vi "SpeedTest.vi"() -> ()   [LabVIEW 2010]
panel:
  out "Numeric":i32
  out "x/y":dbl
  in  "Vi to open":enum16{"JILTest", "JILTest2", "JILTestR"}(ring)
  in  "stringin":string
  in  "booleanin":bool=TRUE
  in  "doublein":dbl
  in  "intin":i32
  in  "Mensajes":T1(ring)
  in  "stop":bool
  in  "Send":bool=TRUE
  out "error out":errorcluster
  out "Respuesta":string
  out "Mensaje":string
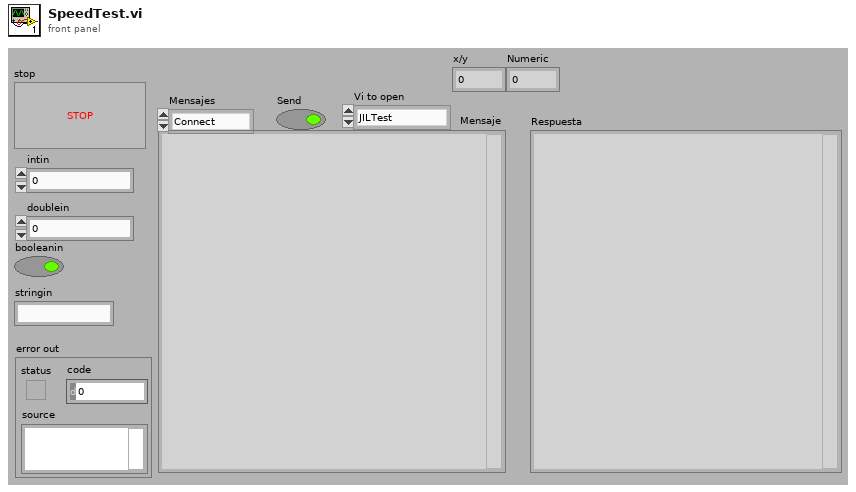
[diagram p1: front panel]
types:
  T1 = enum16{"Connect", "OpenVi", "SyncVi", "RunVi", "StopVi", "CloseVi", "Disconnect"}
  T2 = enum16{"Standard", "Buffered", "CRLF", "Immediate"}
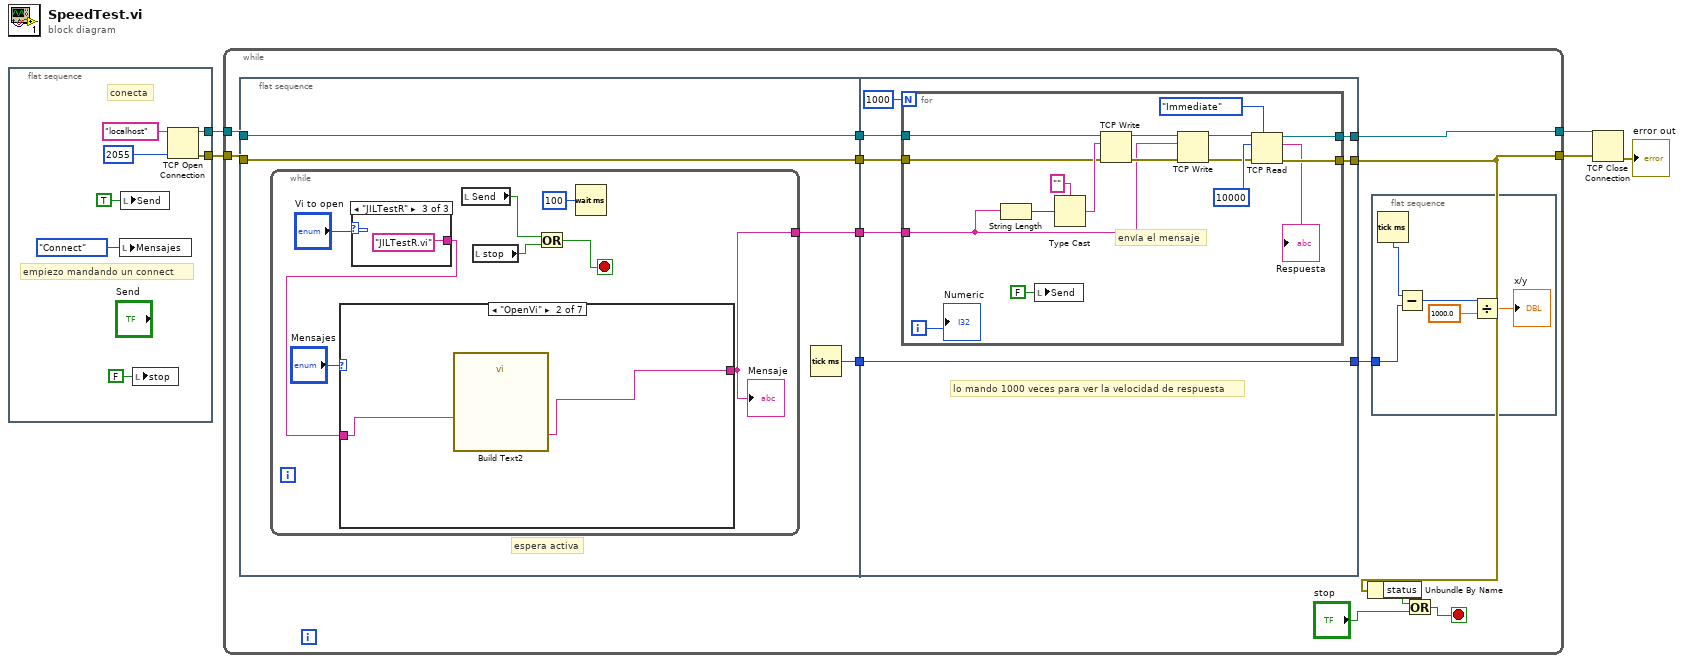
[diagram p0: block diagram]
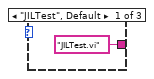
[diagram p2: hidden frame]
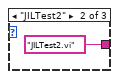
[diagram p3: hidden frame]
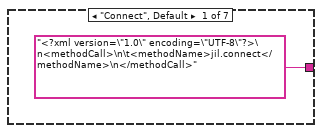
[diagram p4: hidden frame]
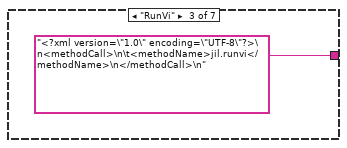
[diagram p5: hidden frame]
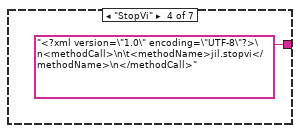
[diagram p6: hidden frame]
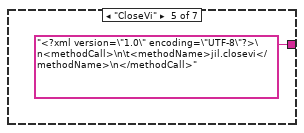
[diagram p7: hidden frame]
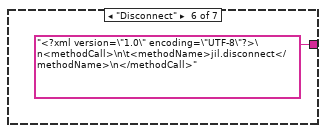
[diagram p8: hidden frame]
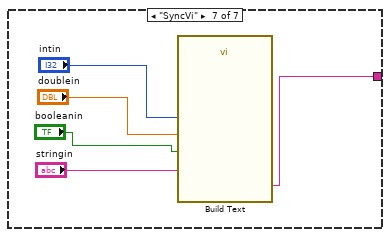
[diagram p9: hidden frame]
diagram:
  n1 = flat-sequence {
    tunnel: [w10] -> w5
    tunnel: [w9] -> w4
    frame #0 {
      # "empiezo mandando un connect"
      # "conecta"
      n2 = local write "Mensajes"(T1."Connect" ("Mensajes")) -> ()
      n3 = local write "Send"(TRUE ("Send")) -> ()
      n4 = local write "stop"(FALSE ("stop")) -> ()
      n5 = TCP Open Connection(address="localhost", remote port or service name=u16 2055) -> (connection ID=w10:refnum<k5>, error out=w9:errorcluster)  [unwired: 3 in]
    }
  }
  n6 = while {
    tunnel: w5 -> [w22]
    tunnel: w4 -> [w21]
    tunnel: [w20] -> w2
    tunnel: [w17] -> w1
    stop <- w18 stop-if-true
    n7 = flat-sequence {
      tunnel: [w33] -> w24
      tunnel: [w32] -> w23
      tunnel: [w31] -> w15
      tunnel: w21 -> [w33]
      tunnel: w22 -> [w32]
      tunnel: [w30] -> w14
      tunnel: [w63] -> w20
      tunnel: [w62] -> w17
      tunnel: w24 -> [w61]
      tunnel: w23 -> [w60]
      tunnel: w15 -> [w59]
      tunnel: [w58] -> w13
      tunnel: w14 -> [w58]
      frame #0 {
        # "espera activa"
        n8 = while {
          tunnel: [w36] -> w31
          stop <- w40 stop-if-true
          n9 = case shown="\"JILTestR\"" "Vi to open" {
            tunnel: ["JILTest.vi" "JILTest2.vi" "JILTestR.vi"] -> w34
            frame "JILTest", Default {
            }
            frame "JILTest2" {
            }
            frame "JILTestR" {
            }
          }
          n10 = case shown="\"OpenVi\"" "Mensajes" {
            tunnel: ["<?xml version=\"1.0\" encoding=\"UTF-8\"?>\n<methodCall>\n\t<methodName>jil.connect</methodName>\n</methodCall>" w46 "<?xml version=\"1.0\" encoding=\"UTF-8\"?>\n<methodCall>\n\t<methodName>jil.runvi</methodName>\n</methodCall>\n" "<?xml version=\"1.0\" encoding=\"UTF-8\"?>\n<methodCall>\n\t<methodName>jil.stopvi</methodName>\n</methodCall>" "<?xml version=\"1.0\" encoding=\"UTF-8\"?>\n<methodCall>\n\t<methodName>jil.closevi</methodName>\n</methodCall>" "<?xml version=\"1.0\" encoding=\"UTF-8\"?>\n<methodCall>\n\t<methodName>jil.disconnect</methodName>\n</methodCall>" w56] -> w36
            tunnel: w34 -> [_ w47 _ _ _ _ _]
            frame "Connect", Default {
            }
            frame "OpenVi" {
              n11 = call "Build Text2"("name"=w47) -> ("Result"=w46:string)  [unwired: 13 in, 1 out]
            }
            frame "RunVi" {
            }
            frame "StopVi" {
            }
            frame "CloseVi" {
            }
            frame "Disconnect" {
            }
            frame "SyncVi" {
              n12 = call "Build Text"("string"="stringin", "int"="intin", "double"="doublein", "bolean"="booleanin") -> ("Result"=w56:string)  [unwired: 10 in, 1 out]
            }
          }
          "Mensaje" <- w36
          n13 = local read "Send"() -> (w38:bool)
          n14 = local read "stop"() -> (w39:bool)
          n15 = Or(x=w38, y=w39) -> (x .or. y?=w40:bool)
          n16 = Wait (ms)(milliseconds to wait=u32 100) -> ()  [unwired: 1 out]
        }
        n17 = Tick Count (ms)() -> (millisecond timer value=w30:u32)
      }
      frame #1 {
        # "lo mando 1000 veces para ver la velocidad de respuesta"
        n18 = for {
          N: 1000 -> [_]
          tunnel: [w71] -> w63
          tunnel: [w70] -> w62
          tunnel: w61 -> [w69]
          tunnel: w60 -> [w68]
          tunnel: w59 -> [w66]
          i -> [w64]
          # "envía el mensaje"
          n19 = String Length(string=w66) -> (length=w74:i32)
          n20 = local write "Send"(FALSE ("Send")) -> ()
          n21 = Type Cast(type="", x=w74) -> (*(type *) &x=w76:string)
          n22 = TCP Write(connection ID=w68, data in=w76, error in (no error)=w69) -> (connection ID out=w72:refnum<k5>, error out=w73:errorcluster)  [unwired: 1 in, 1 out]
          n23 = TCP Write(connection ID=w72, data in=w66, error in (no error)=w73) -> (connection ID out=w77:refnum<k5>, error out=w78:errorcluster)  [unwired: 1 in, 1 out]
          n24 = TCP Read(connection ID=w77, bytes to read=10000, error in (no error)=w78, 7:T2."Immediate" ("mode (standard)")) -> (connection ID out=w71:refnum<k5>, data out=→"Respuesta":string, error out=w70:errorcluster)  [unwired: 1 in]
          "Numeric" <- w64
        }
      }
    }
    n25 = Unbundle By Name(w17) -> ("status"=w16:bool)
    n26 = flat-sequence {
      tunnel: w13 -> [w28]
      frame #0 {
        n27 = Tick Count (ms)() -> (millisecond timer value=w29:u32)
        n28 = Subtract(x=w29, y=w28) -> (x-y=w26:u32)
        n29 = Divide(x=w26, y=1000.0) -> (x/y=→"x/y":dbl)
      }
    }
    n30 = Or(x=w16, y="stop") -> (x .or. y?=w18:bool)
  }
  n31 = TCP Close Connection(connection ID=w2, error in (no error)=w1) -> (error out=→"error out":errorcluster)  [unwired: 1 in, 1 out]
